vi "header data string.vi"(0 "Temperature Control Parameters":T2 {"End Temp" format="%.2f"; "Temp Step" format="%.2f"; "Start Temp" format="%.2f"}, 5 "N temps":i32, 11 "error in (no error)":errorcluster, 13 "Timing Control Parameters":T1 {"Measurment time interval" format="%.2e"}) -> (4 "Header string component":string, 15 "error out":errorcluster)   [LabVIEW 2014]
doc: "From the temperature and control parameters, it returns a header string with lables scorresponding to the data.\n\nBeverly Abadines\nPHY 350\nBAP3B"
uses:
  typedefs/temp control params.ctl
  typedefs/time control params.ctl
panel:
  # "Header Data String Generator"
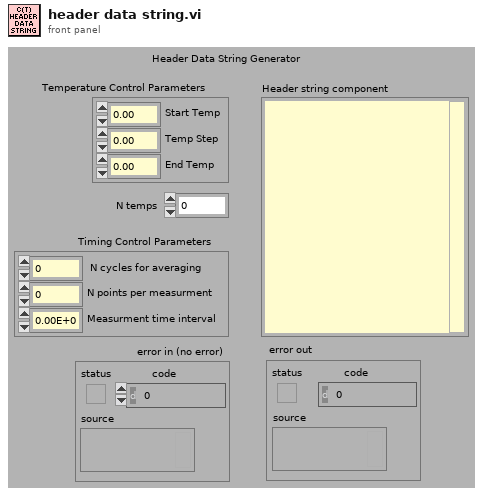
[diagram p1: front panel]
types:
  T1 = typedef "time control params.ctl" = cluster{"N cycles for averaging":i32, "N points per measurment":i32, "Measurment time interval":dbl}
  T2 = typedef "temp control params.ctl" = cluster{"Start Temp":dbl, "Temp Step":dbl, "End Temp":dbl}
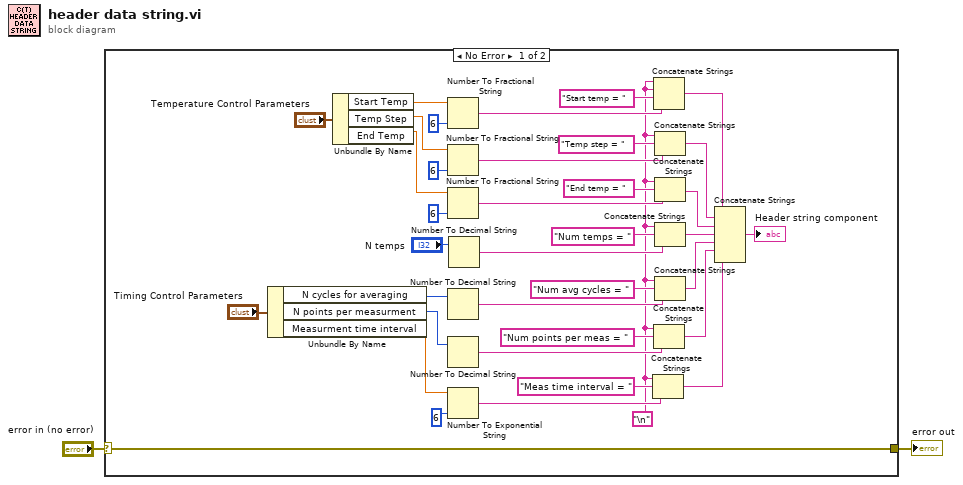
[diagram p0: block diagram]
diagram:
  n1 = case shown="No Error" "error in (no error)" {
    selector: "error in (no error)" -> [w6 w40]
    tunnel: [w6 w40] -> w1
    frame No Error {
      w3 = "\n"
      n2 = Unbundle By Name("Timing Control Parameters") -> ("N cycles for averaging"=w9:i32, "N points per measurment"=w8:i32, "Measurment time interval"=w7:dbl)
      n3 = Unbundle By Name("Temperature Control Parameters") -> ("Start Temp"=w4:dbl, "Temp Step"=w5:dbl, "End Temp"=w11:dbl)
      n4 = Number To Fractional String(number=w4, precision (6)=i16 6) -> (F-format string=w37:string)  [unwired: 2 in]
      n5 = Number To Fractional String(number=w5, precision (6)=i16 6) -> (F-format string=w36:string)  [unwired: 2 in]
      n6 = Number To Fractional String(number=w11, precision (6)=i16 6) -> (F-format string=w35:string)  [unwired: 2 in]
      n7 = Number To Decimal String(number=w9) -> (decimal integer string=w33:string)  [unwired: 1 in]
      n8 = Number To Decimal String(number=w8) -> (decimal integer string=w32:string)  [unwired: 1 in]
      n9 = Number To Exponential String(number=w7, precision (6)=i16 6) -> (E-format string=w31:string)  [unwired: 2 in]
      n10 = Number To Decimal String(number="N temps") -> (decimal integer string=w34:string)  [unwired: 1 in]
      n11 = Concatenate Strings(w3, "Meas time interval = ", w31) -> (w14:string)
      n12 = Concatenate Strings(w3, w3, "Start temp = ", w37) -> (w20:string)
      n13 = Concatenate Strings(w3, "Num points per meas = ", w32) -> (w15:string)
      n14 = Concatenate Strings(w3, "Temp step = ", w36) -> (w19:string)
      n15 = Concatenate Strings(w3, "End temp = ", w35) -> (w18:string)
      n16 = Concatenate Strings(w3, "Num temps = ", w34) -> (w17:string)
      n17 = Concatenate Strings(w3, "Num avg cycles = ", w33) -> (w16:string)
      n18 = Concatenate Strings(w20, w19, w18, w17, w16, w15, w14) -> (→"Header string component":string)
    }
    frame Error {
    }
  }
  "error out" <- w1
